vi "Attempt to close binary refs.vi"(8 "error in (no error)":errorcluster) -> (0 "error out":errorcluster)   [LabVIEW 2013]
uses:
  Functional Imaging Viewer/Typedefs/Get-Set-Clear Control.ctl
  Globals/gl_Time series viewer globals.vi
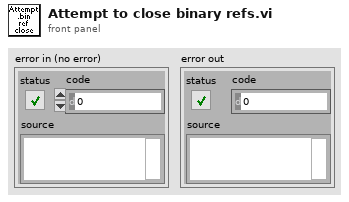
[diagram p1: front panel]
types:
  T1 = typedef "Timelapse viewer refs.ctl" = cluster{"This VI":refnum<vi>, "AVI Mode ind":refnum<vi>, "Play":refnum<vi>, "Stop":refnum<vi>, "Back":refnum<vi>, "Scrollbar":refnum<vi>, "Video length info":refnum<vi>, "Expected speed values":refnum<vi>, "Intensity":refnum<vi>, "Path":refnum<vi>, "Selection sliders":refnum<vi>, "Speed Graph ref":refnum<vi>, "Frame rate set (fps)":refnum<vi>}
  T2 = typedef "Get-Set-Clear Control.ctl" = enum16{"Get", "Set", "Clear"}
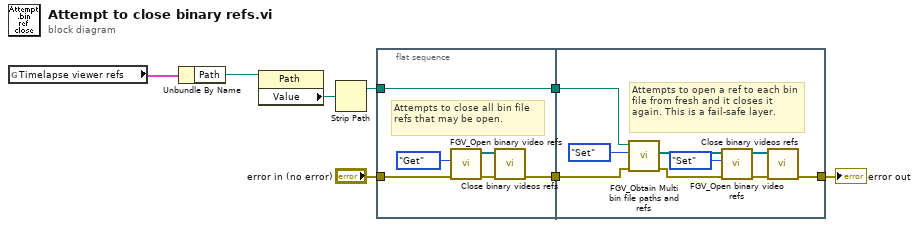
[diagram p0: block diagram]
diagram:
  n1 = global read "gl_Time series viewer globals.vi" "Timelapse viewer refs"() -> (w6:T1)
  n2 = Unbundle By Name(w6) -> ("Path"=w7:refnum<vi>)
  n3 = property class="Path"(reference=w7) -> ("Value"=w8:path)  [unwired: 1 in, 2 out]
  n4 = Strip Path(path=w8) -> (stripped path=w4:path)  [unwired: 1 out]
  n5 = flat-sequence {
    tunnel: w4 -> [w14]
    tunnel: [w14] -> w3
    tunnel: [w10] -> w2
    tunnel: "error in (no error)" -> [w9]
    tunnel: [w23] -> w5
    tunnel: w3 -> [w22]
    tunnel: w2 -> [w15]
    frame #0 {
      # "Attempts to close all bin file refs that may be open."
      n6 = call "FGV_Open binary video refs.vi"("error in (no error)"=w9, "Function"=Get-Set-Clear_Control."Get") -> ("error out"=w13:errorcluster, "Cam Binary Videos (ref)"=w12:refnum<file>[])  [unwired: 8 in]
      n7 = call "Close binary videos refs.vi"("error in"=w13, "Cam Binary Videos"=w12) -> ("error out (no error)"=w10:errorcluster)  [unwired: 9 in]
    }
    frame #1 {
      # "Attempts to open a ref to each bin file from fresh and it closes it again. This is a fail-safe layer."
      n8 = call "FGV_Obtain Multi bin file paths and refs.vi"("error in (no error)"=w15, "Function"=Get-Set-Clear_Control."Set", "Timelapse folder path"=w22) -> ("Error out"=w16:errorcluster, "Cam Binary Videos"=w20:path[])  [unwired: 7 in]
      n9 = call "FGV_Open binary video refs.vi"("error in (no error)"=w16, "Function"=Get-Set-Clear_Control."Set", "Filtered Array in"=w20) -> ("error out"=w19:errorcluster, "Cam Binary Videos (ref)"=w18:refnum<file>[])  [unwired: 7 in]
      n10 = call "Close binary videos refs.vi"("error in"=w19, "Cam Binary Videos"=w18) -> ("error out (no error)"=w23:errorcluster)  [unwired: 9 in]
    }
  }
  "error out" <- w5
